vi "Move.vi"(8 "error in (no error)":errorcluster, 10 "Move Data":cluster{"Direction":T1, "Step (px)":u16}, 11 "PacMan In":refnum<class "PacMan.lvclass">=refnum) -> (0 "error out":errorcluster, 3 "PacMan Out":refnum<class "PacMan.lvclass">)   [LabVIEW 2016, in "PacManClasses.lvlib" / "PacMan.lvclass"]
uses:
  PacMan.lvclass
  C:/Users/lucamach/Documents/SE/Learning OOP/PacMan/PacMan Classes/Geometric Figure/UI Object.lvclass
  Generic Controls/Direction.ctl
  Generic Controls/PacMan Arc.ctl
  Geometric Figure/UI Object.lvclass/UI Object.ctl
  Geometric Figure/Read Center (px).vi
  Geometric Figure/Write Center (px).vi
  PacManClasses.lvlib
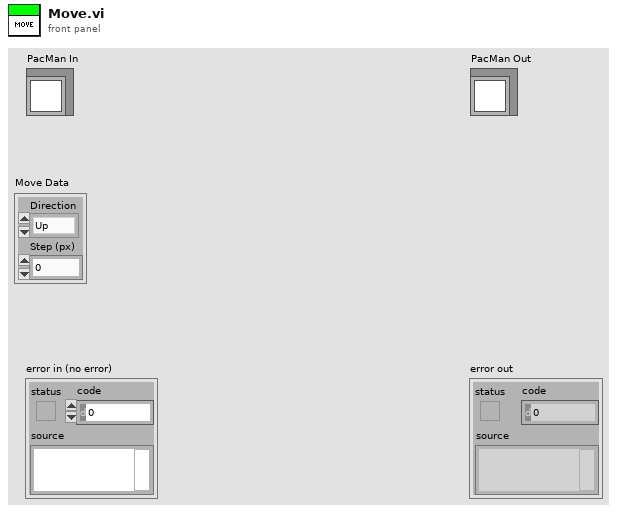
[diagram p1: front panel]
types:
  T1 = typedef "PacManClasses.lvlib/Direction.ctl" = enum16{"Up", "Down", "Left", "Right"}
  T2 = typedef "PacManClasses.lvlib/PacMan Arc.ctl" = cluster{"Start Angle (°)":i16, "Arc Size (°)":i16}
  T3 = typedef "PacManClasses.lvlib/Point.ctl" = cluster{"x":u16, "y":u16}
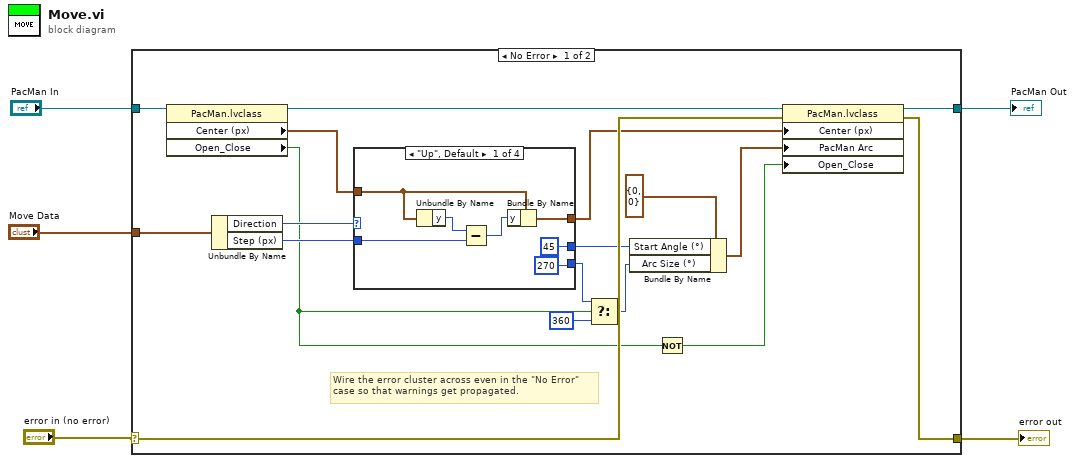
[diagram p0: block diagram]
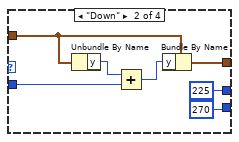
[diagram p2: hidden frame]
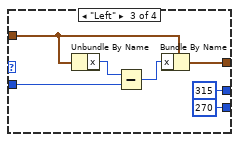
[diagram p3: hidden frame]
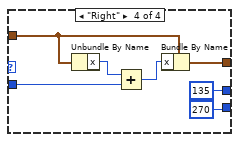
[diagram p4: hidden frame]
diagram:
  n1 = case shown="No Error" "error in (no error)" {
    selector: "error in (no error)" -> [w19 w53]
    tunnel: [w18 w53] -> w4
    tunnel: [w20 w52] -> w1
    tunnel: "PacMan In" -> [w16 w52]
    tunnel: "Move Data" -> [w23 _]
    frame No Error {
      # "Wire the error cluster across even in the \"No Error\"\ncase so that warnings get propagated."
      n2 = property class="PacMan.lvclass"(reference=w16) -> (reference out=w14:refnum<class "PacMan.lvclass">, "Center (px)"=w15:T3, "Open_Close"=w6:bool)  [unwired: 1 in, 1 out]
      n3 = Unbundle By Name(w23) -> ("Direction"=w22:T1, "Step (px)"=w21:u16)
      n4 = case shown="\"Up\", Default" w22 {
        tunnel: w15 -> [w30 w37 w44 w51]
        tunnel: w21 -> [w28 w35 w42 w49]
        tunnel: [w26 w33 w40 w47] -> w17
        tunnel: [i16 45 ("Start Angle (°)") i16 225 ("Start Angle (°)") i16 315 ("Start Angle (°)") i16 135 ("Start Angle (°)")] -> w12
        tunnel: [i16 270 ("Start Angle (°)") i16 270 ("Start Angle (°)") i16 270 ("Start Angle (°)") i16 270 ("Start Angle (°)")] -> w10
        frame "Up", Default {
          n5 = Unbundle By Name(w30) -> ("y"=w29:u16)
          n6 = Subtract(x=w29, y=w28) -> (x-y=w27:u16)
          n7 = Bundle By Name(cluster=w30, "y"=w27) -> (w26:T3)
        }
        frame "Down" {
          n8 = Unbundle By Name(w37) -> ("y"=w36:u16)
          n9 = Add(x=w36, y=w35) -> (x+y=w34:u16)
          n10 = Bundle By Name(cluster=w37, "y"=w34) -> (w33:T3)
        }
        frame "Left" {
          n11 = Unbundle By Name(w44) -> ("x"=w43:u16)
          n12 = Subtract(x=w43, y=w42) -> (x-y=w41:u16)
          n13 = Bundle By Name(cluster=w44, "x"=w41) -> (w40:T3)
        }
        frame "Right" {
          n14 = Unbundle By Name(w51) -> ("x"=w50:u16)
          n15 = Add(x=w50, y=w49) -> (x+y=w48:u16)
          n16 = Bundle By Name(cluster=w51, "x"=w48) -> (w47:T3)
        }
      }
      n17 = Select(t=w10, s=w6, f=i16 360) -> (s? t:f=w8:i16)
      n18 = Bundle By Name(cluster=T2 {"Start Angle (°)"=0, "Arc Size (°)"=0} ("PacMan Arc"), "Start Angle (°)"=w12, "Arc Size (°)"=w8) -> (w11:T2)
      n19 = Not(x=w6) -> (.not. x?=w7:bool)
      n20 = property class="PacMan.lvclass"(reference=w14, error in=w19, "Center (px)"=w17, "PacMan Arc"=w11, "Open_Close"=w7) -> (reference out=w20:refnum<class "PacMan.lvclass">, error out=w18:errorcluster)
    }
    frame Error {
    }
  }
  "error out" <- w4
  "PacMan Out" <- w1
